vi "FipsAdjacent.vi"() -> (11 "Fips":i32[](array[numeric]))   [LabVIEW 2017] (continued)
Municipio, PR\"\t72013\n\"Hatillo Municipio, PR\"\t72065\t\"Camuy Municipio, PR\"\t72027\n\"Hatillo Municipio, PR\"\t72065\t\"Hatillo Municipio, PR\"\t72065\n\"Hatillo Municipio, PR\"\t72065\t\"Lares Municipio, PR\"\t72081\n\"Hatillo Municipio, PR\"\t72065\t\"Utuado Municipio, PR\"\t72141\n\"Hormigueros Municipio, PR\"\t72067\t\"Cabo Rojo Municipio, PR\"\t72023\n\"Hormigueros Municipio, PR\"\t72067\t\"Hormigueros Municipio, PR\"\t72067\n\"Hormigueros Municipio, PR\"\t72067\t\"Mayag?ez Municipio, PR\"\t72097\n\"Hormigueros Municipio, PR\"\t72067\t\"San Germ?n Municipio, PR\"\t72125\n\"Humacao Municipio, PR\"\t72069\t\"Humacao Municipio, PR\"\t72069\n\"Humacao Municipio, PR\"\t72069\t\"Las Piedras Municipio, PR\"\t72085\n\"Humacao Municipio, PR\"\t72069\t\"Naguabo Municipio, PR\"\t72103\n\"Humacao Municipio, PR\"\t72069\t\"Yabucoa Municipio, PR\"\t72151\n\"Isabela Municipio, PR\"\t72071\t\"Aguadilla Municipio, PR\"\t72005\n\"Isabela Municipio, PR\"\t72071\t\"Isabela Municipio, PR\"\t72071\n\"Isabela Municipio, PR\"\t72071\t\"Moca Municipio, PR\"\t72099\n\"Isabela Municipio, PR\"\t72071\t\"Quebradillas Municipio, PR\"\t72115\n\"Isabela Municipio, PR\"\t72071\t\"San Sebasti?n Municipio, PR\"\t72131\n\"Jayuya Municipio, PR\"\t72073\t\"Ciales Municipio, PR\"\t72039\n\"Jayuya Municipio, PR\"\t72073\t\"Jayuya Municipio, PR\"\t72073\n\"Jayuya Municipio, PR\"\t72073\t\"Juana D?az Municipio, PR\"\t72075\n\"Jayuya Municipio, PR\"\t72073\t\"Orocovis Municipio, PR\"\t72107\n\"Jayuya Municipio, PR\"\t72073\t\"Ponce Municipio, PR\"\t72113\n\"Jayuya Municipio, PR\"\t72073\t\"Utuado Municipio, PR\"\t72141\n\"Juana D?az Municipio, PR\"\t72075\t\"Coamo Municipio, PR\"\t72043\n\"Juana D?az Municipio, PR\"\t72075\t\"Jayuya Municipio, PR\"\t72073\n\"Juana D?az Municipio, PR\"\t72075\t\"Juana D?az Municipio, PR\"\t72075\n\"Juana D?az Municipio, PR\"\t72075\t\"Orocovis Municipio, PR\"\t72107\n\"Juana D?az Municipio, PR\"\t72075\t\"Ponce Municipio, PR\"\t72113\n\"Juana D?az Municipio, PR\"\t72075\t\"Santa Isabel Municipio, PR\"\t72133\n\"Juana D?az Municipio, PR\"\t72075\t\"Villalba Municipio, PR\"\t72149\n\"Juncos Municipio, PR\"\t72077\t\"Can?vanas Municipio, PR\"\t72029\n\"Juncos Municipio, PR\"\t72077\t\"Carolina Municipio, PR\"\t72031\n\"Juncos Municipio, PR\"\t72077\t\"Gurabo Municipio, PR\"\t72063\n\"Juncos Municipio, PR\"\t72077\t\"Juncos Municipio, PR\"\t72077\n\"Juncos Municipio, PR\"\t72077\t\"Las Piedras Municipio, PR\"\t72085\n\"Juncos Municipio, PR\"\t72077\t\"San Lorenzo Municipio, PR\"\t72129\n\"Lajas Municipio, PR\"\t72079\t\"Cabo Rojo Municipio, PR\"\t72023\n\"Lajas Municipio, PR\"\t72079\t\"Gu?nica Municipio, PR\"\t72055\n\"Lajas Municipio, PR\"\t72079\t\"Lajas Municipio, PR\"\t72079\n\"Lajas Municipio, PR\"\t72079\t\"Sabana Grande Municipio, PR\"\t72121\n\"Lajas Municipio, PR\"\t72079\t\"San Germ?n Municipio, PR\"\t72125\n\"Lares Municipio, PR\"\t72081\t\"Adjuntas Municipio, PR\"\t72001\n\"Lares Municipio, PR\"\t72081\t\"Camuy Municipio, PR\"\t72027\n\"Lares Municipio, PR\"\t72081\t\"Hatillo Municipio, PR\"\t72065\n\"Lares Municipio, PR\"\t72081\t\"Lares Municipio, PR\"\t72081\n\"Lares Municipio, PR\"\t72081\t\"Las Mar?as Municipio, PR\"\t72083\n\"Lares Municipio, PR\"\t72081\t\"Maricao Municipio, PR\"\t72093\n\"Lares Municipio, PR\"\t72081\t\"San Sebasti?n Municipio, PR\"\t72131\n\"Lares Municipio, PR\"\t72081\t\"Utuado Municipio, PR\"\t72141\n\"Lares Municipio, PR\"\t72081\t\"Yauco Municipio, PR\"\t72153\n\"Las Mar?as Municipio, PR\"\t72083\t\"A?asco Municipio, PR\"\t72011\n\"Las Mar?as Municipio, PR\"\t72083\t\"Lares Municipio, PR\"\t72081\n\"Las Mar?as Municipio, PR\"\t72083\t\"Las Mar?as Municipio, PR\"\t72083\n\"Las Mar?as Municipio, PR\"\t72083\t\"Maricao Municipio, PR\"\t72093\n\"Las Mar?as Municipio, PR\"\t72083\t\"Mayag?ez Municipio, PR\"\t72097\n\"Las Mar?as Municipio, PR\"\t72083\t\"San Sebasti?n Municipio, PR\"\t72131\n\"Las Piedras Municipio, PR\"\t72085\t\"Can?vanas Municipio, PR\"\t72029\n\"Las Piedras Municipio, PR\"\t72085\t\"Humacao Municipio, PR\"\t72069\n\"Las Piedras Municipio, PR\"\t72085\t\"Juncos Municipio, PR\"\t72077\n\"Las Piedras Municipio, PR\"\t72085\t\"Las Piedras Municipio, PR\"\t72085\n\"Las Piedras Municipio, PR\"\t72085\t\"Naguabo Municipio, PR\"\t72103\n\"Las Piedras Municipio, PR\"\t72085\t\"R?o Grande Municipio, PR\"\t72119\n\"Las Piedras Municipio, PR\"\t72085\t\"San Lorenzo Municipio, PR\"\t72129\n\"Las Piedras Municipio, PR\"\t72085\t\"Yabucoa Municipio, PR\"\t72151\n\"Lo?za Municipio, PR\"\t72087\t\"Can?vanas Municipio, PR\"\t72029\n\"Lo?za Municipio, PR\"\t72087\t\"Carolina Municipio, PR\"\t72031\n\"Lo?za Municipio, PR\"\t72087\t\"Lo?za Municipio, PR\"\t72087\n\"Lo?za Municipio, PR\"\t72087\t\"R?o Grande Municipio, PR\"\t72119\n\"Luquillo Municipio, PR\"\t72089\t\"Ceiba Municipio, PR\"\t72037\n\"Luquillo Municipio, PR\"\t72089\t\"Fajardo Municipio, PR\"\t72053\n\"Luquillo Municipio, PR\"\t72089\t\"Luquillo Municipio, PR\"\t72089\n\"Luquillo Municipio, PR\"\t72089\t\"R?o Grande Municipio, PR\"\t72119\n\"Manat? Municipio, PR\"\t72091\t\"Barceloneta Municipio, PR\"\t72017\n\"Manat? Municipio, PR\"\t72091\t\"Ciales Municipio, PR\"\t72039\n\"Manat? Municipio, PR\"\t72091\t\"Florida Municipio, PR\"\t72054\n\"Manat? Municipio, PR\"\t72091\t\"Manat? Municipio, PR\"\t72091\n\"Manat? Municipio, PR\"\t72091\t\"Morovis Municipio, PR\"\t72101\n\"Manat? Municipio, PR\"\t72091\t\"Vega Alta Municipio, PR\"\t72143\n\"Manat? Municipio, PR\"\t72091\t\"Vega Baja Municipio, PR\"\t72145\n\"Maricao Municipio, PR\"\t72093\t\"Lares Municipio, PR\"\t72081\n\"Maricao Municipio, PR\"\t72093\t\"Las Mar?as Municipio, PR\"\t72083\n\"Maricao Municipio, PR\"\t72093\t\"Maricao Municipio, PR\"\t72093\n\"Maricao Municipio, PR\"\t72093\t\"Mayag?ez Municipio, PR\"\t72097\n\"Maricao Municipio, PR\"\t72093\t\"Sabana Grande Municipio, PR\"\t72121\n\"Maricao Municipio, PR\"\t72093\t\"San Germ?n Municipio, PR\"\t72125\n\"Maricao Municipio, PR\"\t72093\t\"Yauco Municipio, PR\"\t72153\n\"Maunabo Municipio, PR\"\t72095\t\"Maunabo Municipio, PR\"\t72095\n\"Maunabo Municipio, PR\"\t72095\t\"Patillas Municipio, PR\"\t72109\n\"Maunabo Municipio, PR\"\t72095\t\"Yabucoa Municipio, PR\"\t72151\n\"Mayag?ez Municipio, PR\"\t72097\t\"A?asco Municipio, PR\"\t72011\n\"Mayag?ez Municipio, PR\"\t72097\t\"Cabo Rojo Municipio, PR\"\t72023\n\"Mayag?ez Municipio, PR\"\t72097\t\"Hormigueros Municipio, PR\"\t72067\n\"Mayag?ez Municipio, PR\"\t72097\t\"Las Mar?as Municipio, PR\"\t72083\n\"Mayag?ez Municipio, PR\"\t72097\t\"Maricao Municipio, PR\"\t72093\n\"Mayag?ez Municipio, PR\"\t72097\t\"Mayag?ez Municipio, PR\"\t72097\n\"Mayag?ez Municipio, PR\"\t72097\t\"Rinc?n Municipio, PR\"\t72117\n\"Mayag?ez Municipio, PR\"\t72097\t\"San Germ?n Municipio, PR\"\t72125\n\"Moca Municipio, PR\"\t72099\t\"Aguada Municipio, PR\"\t72003\n\"Moca Municipio, PR\"\t72099\t\"Aguadilla Municipio, PR\"\t72005\n\"Moca Municipio, PR\"\t72099\t\"A?asco Municipio, PR\"\t72011\n\"Moca Municipio, PR\"\t72099\t\"Isabela Municipio, PR\"\t72071\n\"Moca Municipio, PR\"\t72099\t\"Moca Municipio, PR\"\t72099\n\"Moca Municipio, PR\"\t72099\t\"San Sebasti?n Municipio, PR\"\t72131\n\"Morovis Municipio, PR\"\t72101\t\"Ciales Municipio, PR\"\t72039\n\"Morovis Municipio, PR\"\t72101\t\"Corozal Municipio, PR\"\t72047\n\"Morovis Municipio, PR\"\t72101\t\"Manat? Municipio, PR\"\t72091\n\"Morovis Municipio, PR\"\t72101\t\"Morovis Municipio, PR\"\t72101\n\"Morovis Municipio, PR\"\t72101\t\"Orocovis Municipio, PR\"\t72107\n\"Morovis Municipio, PR\"\t72101\t\"Vega Alta Municipio, PR\"\t72143\n\"Morovis Municipio, PR\"\t72101\t\"Vega Baja Municipio, PR\"\t72145\n\"Naguabo Municipio, PR\"\t72103\t\"Ceiba Municipio, PR\"\t72037\n\"Naguabo Municipio, PR\"\t72103\t\"Humacao Municipio, PR\"\t72069\n\"Naguabo Municipio, PR\"\t72103\t\"Las Piedras Municipio, PR\"\t72085\n\"Naguabo Municipio, PR\"\t72103\t\"Naguabo Municipio, PR\"\t72103\n\"Naguabo Municipio, PR\"\t72103\t\"R?o Grande Municipio, PR\"\t72119\n\"Naranjito Municipio, PR\"\t72105\t\"Barranquitas Municipio, PR\"\t72019\n\"Naranjito Municipio, PR\"\t72105\t\"Bayam?n Municipio, PR\"\t72021\n\"Naranjito Municipio, PR\"\t72105\t\"Comer?o Municipio, PR\"\t72045\n\"Naranjito Municipio, PR\"\t72105\t\"Corozal Municipio, PR\"\t72047\n\"Naranjito Municipio, PR\"\t72105\t\"Naranjito Municipio, PR\"\t72105\n\"Naranjito Municipio, PR\"\t72105\t\"Toa Alta Municipio, PR\"\t72135\n\"Orocovis Municipio, PR\"\t72107\t\"Barranquitas Municipio, PR\"\t72019\n\"Orocovis Municipio, PR\"\t72107\t\"Ciales Municipio, PR\"\t72039\n\"Orocovis Municipio, PR\"\t72107\t\"Coamo Municipio, PR\"\t72043\n\"Orocovis Municipio, PR\"\t72107\t\"Corozal Municipio, PR\"\t72047\n\"Orocovis Municipio, PR\"\t72107\t\"Jayuya Municipio, PR\"\t72073\n\"Orocovis Municipio, PR\"\t72107\t\"Juana D?az Municipio, PR\"\t72075\n\"Orocovis Municipio, PR\"\t72107\t\"Morovis Municipio, PR\"\t72101\n\"Orocovis Municipio, PR\"\t72107\t\"Orocovis Municipio, PR\"\t72107\n\"Orocovis Municipio, PR\"\t72107\t\"Villalba Municipio, PR\"\t72149\n\"Patillas Municipio, PR\"\t72109\t\"Arroyo Municipio, PR\"\t72015\n\"Patillas Municipio, PR\"\t72109\t\"Cayey Municipio, PR\"\t72035\n\"Patillas Municipio, PR\"\t72109\t\"Guayama Municipio, PR\"\t72057\n\"Patillas Municipio, PR\"\t72109\t\"Maunabo Municipio, PR\"\t72095\n\"Patillas Municipio, PR\"\t72109\t\"Patillas Municipio, PR\"\t72109\n\"Patillas Municipio, PR\"\t72109\t\"San Lorenzo Municipio, PR\"\t72129\n\"Patillas Municipio, PR\"\t72109\t\"Yabucoa Municipio, PR\"\t72151\n\"Pe?uelas Municipio, PR\"\t72111\t\"Adjuntas Municipio, PR\"\t72001\n\"Pe?uelas Municipio, PR\"\t72111\t\"Guayanilla Municipio, PR\"\t72059\n\"Pe?uelas Municipio, PR\"\t72111\t\"Pe?uelas Municipio, PR\"\t72111\n\"Pe?uelas Municipio, PR\"\t72111\t\"Ponce Municipio, PR\"\t72113\n\"Ponce Municipio, PR\"\t72113\t\"Adjuntas Municipio, PR\"\t72001\n\"Ponce Municipio, PR\"\t72113\t\"Jayuya Municipio, PR\"\t72073\n\"Ponce Municipio, PR\"\t72113\t\"Juana D?az Municipio, PR\"\t72075\n\"Ponce Municipio, PR\"\t72113\t\"Pe?uelas Municipio, PR\"\t72111\n\"Ponce Municipio, PR\"\t72113\t\"Ponce Municipio, PR\"\t72113\n\"Ponce Municipio, PR\"\t72113\t\"Utuado Municipio, PR\"\t72141\n\"Quebradillas Municipio, PR\"\t72115\t\"Camuy Municipio, PR\"\t72027\n\"Quebradillas Municipio, PR\"\t72115\t\"Isabela Municipio, PR\"\t72071\n\"Quebradillas Municipio, PR\"\t72115\t\"Quebradillas Municipio, PR\"\t72115\n\"Quebradillas Municipio, PR\"\t72115\t\"San Sebasti?n Municipio, PR\"\t72131\n\"Rinc?n Municipio, PR\"\t72117\t\"Aguada Municipio, PR\"\t72003\n\"Rinc?n Municipio, PR\"\t72117\t\"A?asco Municipio, PR\"\t72011\n\"Rinc?n Municipio, PR\"\t72117\t\"Mayag?ez Municipio, PR\"\t72097\n\"Rinc?n Municipio, PR\"\t72117\t\"Rinc?n Municipio, PR\"\t72117\n\"R?o Grande Municipio, PR\"\t72119\t\"Can?vanas Municipio, PR\"\t72029\n\"R?o Grande Municipio, PR\"\t72119\t\"Ceiba Municipio, PR\"\t72037\n\"R?o Grande Municipio, PR\"\t72119\t\"Las Piedras Municipio, PR\"\t72085\n\"R?o Grande Municipio, PR\"\t72119\t\"Lo?za Municipio, PR\"\t72087\n\"R?o Grande Municipio, PR\"\t72119\t\"Luquillo Municipio, PR\"\t72089\n\"R?o Grande Municipio, PR\"\t72119\t\"Naguabo Municipio, PR\"\t72103\n\"R?o Grande Municipio, PR\"\t72119\t\"R?o Grande Municipio, PR\"\t72119\n\"Sabana Grande Municipio, PR\"\t72121\t\"Gu?nica Municipio, PR\"\t72055\n\"Sabana Grande Municipio, PR\"\t72121\t\"Lajas Municipio, PR\"\t72079\n\"Sabana Grande Municipio, PR\"\t72121\t\"Maricao Municipio, PR\"\t72093\n\"Sabana Grande Municipio, PR\"\t72121\t\"Sabana Grande Municipio, PR\"\t72121\n\"Sabana Grande Municipio, PR\"\t72121\t\"San Germ?n Municipio, PR\"\t72125\n\"Sabana Grande Municipio, PR\"\t72121\t\"Yauco Municipio, PR\"\t72153\n\"Salinas Municipio, PR\"\t72123\t\"Aibonito Municipio, PR\"\t72009\n\"Salinas Municipio, PR\"\t72123\t\"Cayey Municipio, PR\"\t72035\n\"Salinas Municipio, PR\"\t72123\t\"Coamo Municipio, PR\"\t72043\n\"Salinas Municipio, PR\"\t72123\t\"Guayama Municipio, PR\"\t72057\n\"Salinas Municipio, PR\"\t72123\t\"Salinas Municipio, PR\"\t72123\n\"Salinas Municipio, PR\"\t72123\t\"Santa Isabel Municipio, PR\"\t72133\n\"San Germ?n Municipio, PR\"\t72125\t\"Cabo Rojo Municipio, PR\"\t72023\n\"San Germ?n Municipio, PR\"\t72125\t\"Hormigueros Municipio, PR\"\t72067\n\"San Germ?n Municipio, PR\"\t72125\t\"Lajas Municipio, PR\"\t72079\n\"San Germ?n Municipio, PR\"\t72125\t\"Maricao Municipio, PR\"\t72093\n\"San Germ?n Municipio, PR\"\t72125\t\"Mayag?ez Municipio, PR\"\t72097\n\"San Germ?n Municipio, PR\"\t72125\t\"Sabana Grande Municipio, PR\"\t72121\n\"San Germ?n Municipio, PR\"\t72125\t\"San Germ?n Municipio, PR\"\t72125\n\"San Juan Municipio, PR\"\t72127\t\"Aguas Buenas Municipio, PR\"\t72007\n\"San Juan Municipio, PR\"\t72127\t\"Caguas Municipio, PR\"\t72025\n\"San Juan Municipio, PR\"\t72127\t\"Carolina Municipio, PR\"\t72031\n\"San Juan Municipio, PR\"\t72127\t\"Cata?o Municipio, PR\"\t72033\n\"San Juan Municipio, PR\"\t72127\t\"Guaynabo Municipio, PR\"\t72061\n\"San Juan Municipio, PR\"\t72127\t\"San Juan Municipio, PR\"\t72127\n\"San Juan Municipio, PR\"\t72127\t\"Toa Baja Municipio, PR\"\t72137\n\"San Juan Municipio, PR\"\t72127\t\"Trujillo Alto Municipio, PR\"\t72139\n\"San Lorenzo Municipio, PR\"\t72129\t\"Caguas Municipio, PR\"\t72025\n\"San Lorenzo Municipio, PR\"\t72129\t\"Cayey Municipio, PR\"\t72035\n\"San Lorenzo Municipio, PR\"\t72129\t\"Gurabo Municipio, PR\"\t72063\n\"San Lorenzo Municipio, PR\"\t72129\t\"Juncos Municipio, PR\"\t72077\n\"San Lorenzo Municipio, PR\"\t72129\t\"Las Piedras Municipio, PR\"\t72085\n\"San Lorenzo Municipio, PR\"\t72129\t\"Patillas Municipio, PR\"\t72109\n\"San Lorenzo Municipio, PR\"\t72129\t\"San Lorenzo Municipio, PR\"\t72129\n\"San Lorenzo Municipio, PR\"\t72129\t\"Yabucoa Municipio, PR\"\t72151\n\"San Sebasti?n Municipio, PR\"\t72131\t\"A?asco Municipio, PR\"\t72011\n\"San Sebasti?n Municipio, PR\"\t72131\t\"Camuy Municipio, PR\"\t72027\n\"San Sebasti?n Municipio, PR\"\t72131\t\"Isabela Municipio, PR\"\t72071\n\"San Sebasti?n Municipio, PR\"\t72131\t\"Lares Municipio, PR\"\t72081\n\"San Sebasti?n Municipio, PR\"\t72131\t\"Las Mar?as Municipio, PR\"\t72083\n\"San Sebasti?n Municipio, PR\"\t72131\t\"Moca Municipio, PR\"\t72099\n\"San Sebasti?n Municipio, PR\"\t72131\t\"Quebradillas Municipio, PR\"\t72115\n\"San Sebasti?n Municipio, PR\"\t72131\t\"San Sebasti?n Municipio, PR\"\t72131\n\"Santa Isabel Municipio, PR\"\t72133\t\"Coamo Municipio, PR\"\t72043\n\"Santa Isabel Municipio, PR\"\t72133\t\"Juana D?az Municipio, PR\"\t72075\n\"Santa Isabel Municipio, PR\"\t72133\t\"Salinas Municipio, PR\"\t72123\n\"Santa Isabel Municipio, PR\"\t72133\t\"Santa Isabel Municipio, PR\"\t72133\n\"Toa Alta Municipio, PR\"\t72135\t\"Bayam?n Municipio, PR\"\t72021\n\"Toa Alta Municipio, PR\"\t72135\t\"Corozal Municipio, PR\"\t72047\n\"Toa Alta Municipio, PR\"\t72135\t\"Dorado Municipio, PR\"\t72051\n\"Toa Alta Municipio, PR\"\t72135\t\"Naranjito Municipio, PR\"\t72105\n\"Toa Alta Municipio, PR\"\t72135\t\"Toa Alta Municipio, PR\"\t72135\n\"Toa Alta Municipio, PR\"\t72135\t\"Toa Baja Municipio, PR\"\t72137\n\"Toa Alta Municipio, PR\"\t72135\t\"Vega Alta Municipio, PR\"\t72143\n\"Toa Baja Municipio, PR\"\t72137\t\"Bayam?n Municipio, PR\"\t72021\n\"Toa Baja Municipio, PR\"\t72137\t\"Cata?o Municipio, PR\"\t72033\n\"Toa Baja Municipio, PR\"\t72137\t\"Dorado Municipio, PR\"\t72051\n\"Toa Baja Municipio, PR\"\t72137\t\"San Juan Municipio, PR\"\t72127\n\"Toa Baja Municipio, PR\"\t72137\t\"Toa Alta Municipio, PR\"\t72135\n\"Toa Baja Municipio, PR\"\t72137\t\"Toa Baja Municipio, PR\"\t72137\n\"Trujillo Alto Municipio, PR\"\t72139\t\"Caguas Municipio, PR\"\t72025\n\"Trujillo Alto Municipio, PR\"\t72139\t\"Carolina Municipio, PR\"\t72031\n\"Trujillo Alto Municipio, PR\"\t72139\t\"Gurabo Municipio, PR\"\t72063\n\"Trujillo Alto Municipio, PR\"\t72139\t\"San Juan Municipio, PR\"\t72127\n\"Trujillo Alto Municipio, PR\"\t72139\t\"Trujillo Alto Municipio, PR\"\t72139\n\"Utuado Municipio, PR\"\t72141\t\"Adjuntas Municipio, PR\"\t72001\n\"Utuado Municipio, PR\"\t72141\t\"Arecibo Municipio, PR\"\t72013\n\"Utuado Municipio, PR\"\t72141\t\"Ciales Municipio, PR\"\t72039\n\"Utuado Municipio, PR\"\t72141\t\"Hatillo Municipio, PR\"\t72065\n\"Utuado Municipio, PR\"\t72141\t\"Jayuya Municipio, PR\"\t72073\n\"Utuado Municipio, PR\"\t72141\t\"Lares Municipio, PR\"\t72081\n\"Utuado Municipio, PR\"\t72141\t\"Ponce Municipio, PR\"\t72113\n\"Utuado Municipio, PR\"\t72141\t\"Utuado Municipio, PR\"\t72141\n\"Vega Alta Municipio, PR\"\t72143\t\"Corozal Municipio, PR\"\t72047\n\"Vega Alta Municipio, PR\"\t72143\t\"Dorado Municipio, PR\"\t72051\n\"Vega Alta Municipio, PR\"\t72143\t\"Manat? Municipio, PR\"\t72091\n\"Vega Alta Municipio, PR\"\t72143\t\"Morovis Municipio, PR\"\t72101\n\"Vega Alta Municipio, PR\"\t72143\t\"Toa Alta Municipio, PR\"\t72135\n\"Vega Alta Municipio, PR\"\t72143\t\"Vega Alta Municipio, PR\"\t72143\n\"Vega Alta Municipio, PR\"\t72143\t\"Vega Baja Municipio, PR\"\t72145\n\"Vega Baja Municipio, PR\"\t72145\t\"Manat? Municipio, PR\"\t72091\n\"Vega Baja Municipio, PR\"\t72145\t\"Morovis Municipio, PR\"\t72101\n\"Vega Baja Municipio, PR\"\t72145\t\"Vega Alta Municipio, PR\"\t72143\n\"Vega Baja Municipio, PR\"\t72145\t\"Vega Baja Municipio, PR\"\t72145\n\"Vieques Municipio, PR\"\t72147\t\"Ceiba Municipio, PR\"\t72037\n\"Vieques Municipio, PR\"\t72147\t\"Vieques Municipio, PR\"\t72147\n\"Villalba Municipio, PR\"\t72149\t\"Coamo Municipio, PR\"\t72043\n\"Villalba Municipio, PR\"\t72149\t\"Juana D?az Municipio, PR\"\t72075\n\"Villalba Municipio, PR\"\t72149\t\"Orocovis Municipio, PR\"\t72107\n\"Villalba Municipio, PR\"\t72149\t\"Villalba Municipio, PR\"\t72149\n\"Yabucoa Municipio, PR\"\t72151\t\"Humacao Municipio, PR\"\t72069\n\"Yabucoa Municipio, PR\"\t72151\t\"Las Piedras Municipio, PR\"\t72085\n\"Yabucoa Municipio, PR\"\t72151\t\"Maunabo Municipio, PR\"\t72095\n\"Yabucoa Municipio, PR\"\t72151\t\"Patillas Municipio, PR\"\t72109\n\"Yabucoa Municipio, PR\"\t72151\t\"San Lorenzo Municipio, PR\"\t72129\n\"Yabucoa Municipio, PR\"\t72151\t\"Yabucoa Municipio, PR\"\t72151\n\"Yauco Municipio, PR\"\t72153\t\"Adjuntas Municipio, PR\"\t72001\n\"Yauco Municipio, PR\"\t72153\t\"Gu?nica Municipio, PR\"\t72055\n\"Yauco Municipio, PR\"\t72153\t\"Guayanilla Municipio, PR\"\t72059\n\"Yauco Municipio, PR\"\t72153\t\"Lares Municipio, PR\"\t72081\n\"Yauco Municipio, PR\"\t72153\t\"Maricao Municipio, PR\"\t72093\n\"Yauco Municipio, PR\"\t72153\t\"Sabana Grande Municipio, PR\"\t72121\n\"Yauco Municipio, PR\"\t72153\t\"Yauco Municipio, PR\"\t72153\n\"Eastern District, AS\"\t60010\t\"Eastern District, AS\"\t60010\n\"Eastern District, AS\"\t60010\t\"Western District, AS\"\t60050\n\"Manu'a District, AS\"\t60020\t\"Manu'a District, AS\"\t60020\n\"Rose Island, AS\"\t60030\t\"Rose Island, AS\"\t60030\n\"Swains Island, AS\"\t60040\t\"Swains Island, AS\"\t60040\n\"Western District, AS\"\t60050\t\"Eastern District, AS\"\t60010\n\"Western District, AS\"\t60050\t\"Western District, AS\"\t60050\n\"Guam, GU\"\t66010\t\"Guam, GU\"\t66010\n\"Northern Islands Municipality, MP\"\t69085\t\"Northern Islands Municipality, MP\"\t69085\n\"Rota Municipality, MP\"\t69100\t\"Rota Municipality, MP\"\t69100\n\"Saipan Municipality, MP\"\t69110\t\"Saipan Municipality, MP\"\t69110\n\"Saipan Municipality, MP\"\t69110\t\"Tinian Municipality, MP\"\t69120\n\"Tinian Municipality, MP\"\t69120\t\"Saipan Municipality, MP\"\t69110\n\"Tinian Municipality, MP\"\t69120\t\"Tinian Municipality, MP\"\t69120\n\"St. Croix Island, VI\"\t78010\t\"St. Croix Island, VI\"\t78010\n\"St. John Island, VI\"\t78020\t\"St. John Island, VI\"\t78020\n\"St. John Island, VI\"\t78020\t\"St. Thomas Island, VI\"\t78030\n\"St. Thomas Island, VI\"\t78030\t\"St. John Island, VI\"\t78020\n\"St. Thomas Island, VI\"\t78030\t\"St. Thomas Island, VI\"\t78030\n", array type (2D Dbl)=string[][] []) -> (array=w14:string[][])  [unwired: 1 in]
  n2 = Index Array(array=w14, index (col) #1=0 ("disabled index (col)"), index (col) #2=1 ("index (col)"), index (col) #3=2 ("index (col)"), index (col) #4=3 ("index (col)")) -> (element #2=w10:string[], element #4=w12:string[])  [unwired: 4 in, 2 out]
  n3 = Decimal String To Number(string=w12) -> (number=w3:i32[])  [unwired: 2 in, 1 out]
  "FipsAdj" <- w3
  n4 = Decimal String To Number(string=w10) -> (number=w9:i32[])  [unwired: 2 in, 1 out]
  "Fips" <- w9
  n5 = Delete From Array(array=w9, length=1, index=0) -> (deleted portion=w6:i32[], array with subset deleted=w5:i32[])
  n6 = Index Array(array=w6) -> (element=w4:i32)  [unwired: 1 in]
  n7 = for {
    shift-right: [w28] -> _
    shift-left: w4 -> [w23]
    tunnel: w5 -> [w28] mode=indexing
    shift-right: [w24] -> _
    shift-left: 0 -> [w26]
    tunnel: w3 -> [w27]
    tunnel: [w22] -> w1 mode=indexing if=w20
    i -> [w25]
    n8 = Equal?(x=w28, y=w23) -> (x = y?=w21:bool)
    n9 = case shown="False" w21 {
      tunnel: w27 -> [w36 _]
      tunnel: w26 -> [w34 w37]
      tunnel: w25 -> [w30 _]
      tunnel: [w29 w37] -> w24
      tunnel: w23 -> [w33 _]
      tunnel: [w31 _] -> w22
      frame False {
        n10 = Subtract(x=w30, y=w34) -> (x-y=w35:i32)
        n11 = Array Subset(array=w36, index=w34, length=w35) -> (w32:i32[])
        n12 = Increment(x=w30) -> (x+1=w29:i32)
        n13 = Bundle(w33, w32) -> (w31:cluster{i32, i32[]})  [unwired: 1 in]
      }
      frame True {
      }
    }
    n14 = Not(x=w21) -> (.not. x?=w20:bool)
  }
  "Adjaceny" <- w1
